vi "flattenToString.vi"(8 "error in (no error)":errorcluster, 11 "Task Status in":refnum<class "Task Status.lvclass">) -> (0 "error out":errorcluster, 3 "data string":string)   [LabVIEW 2017, in "Message Interface.lvlib" / "Task Status.lvclass"]
uses:
  Task Status.lvclass
  C:/Users/Public/Documents/wc/BuildFarm/src/LabVIEW/vi.lib/BenjaminR/Build Farm/Classes/Message Interface/Status/Status.lvclass
  Status/Status.lvclass/Status.ctl
  Status/Read Item Name.vi
  Status/Write Item Name.vi
  Status/Status.lvclass
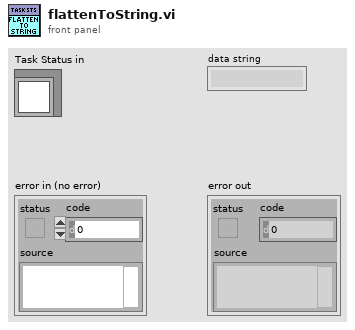
[diagram p1: front panel]
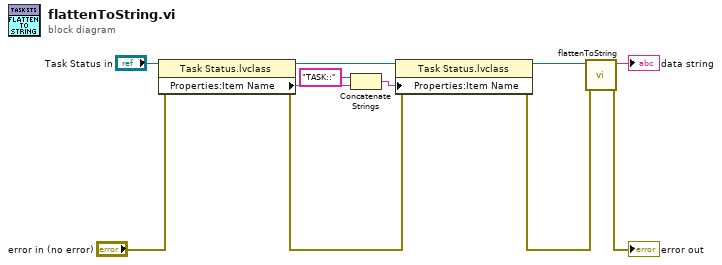
[diagram p0: block diagram]
diagram:
  n1 = property class="Task Status.lvclass"(reference="Task Status in", error in="error in (no error)") -> (reference out=w9:refnum<class "Task Status.lvclass">, error out=w4:errorcluster, "Properties:Item Name"=w7:string)
  n2 = Concatenate Strings("TASK::" ("string"), w7) -> (w8:string)
  n3 = property class="Task Status.lvclass"(reference=w9, error in=w4, "Properties:Item Name"=w8) -> (reference out=w3:refnum<class "Task Status.lvclass">, error out=w1:errorcluster)
  n4 = call-parent "flattenToString.vi"("error in (no error)"=w1, "iMessage in"=w3) -> ("error out"=→"error out":errorcluster, "data string"=→"data string":string)  [unwired: 8 in]
